vi "Secondary Ball Management and Shoot.vi"   [LabVIEW 2011]
uses:
  Team Code/Robot Global Data.vi
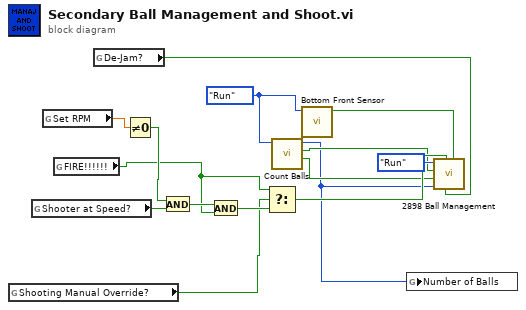
[diagram p0: block diagram]
diagram:
  w1 = enum16{"Init", "Run", "End"}."Run" ("Enum")
  n1 = global read "Robot Global Data.vi" "Shooting Manual Override?"() -> (w9:bool)
  n2 = global read "Robot Global Data.vi" "Shooter at Speed?"() -> (w15:bool)
  n3 = global read "Robot Global Data.vi" "Set RPM"() -> (w12:dbl)
  n4 = global read "Robot Global Data.vi" "FIRE!!!!!!"() -> (w10:bool)
  n5 = global read "Robot Global Data.vi" "De-Jam?"() -> (w3:bool)
  n6 = Not Equal To 0?(x=w12) -> (x != 0?=w11:bool)
  n7 = And(x=w11, y=w15) -> (x .and. y?=w14:bool)
  n8 = And(x=w14, y=w10) -> (x .and. y?=w13:bool)
  n9 = Select(t=w10, s=w9, f=w13) -> (s? t:f=w8:bool)
  n10 = call "Count Balls.vi"("Mode"=w1) -> ("Top Sensor?"=w5:bool, "Bottom Back?"=w6:bool, "Number Of Balls"=w4:i32)  [unwired: 8 in]
  n11 = call "Bottom Front Sensor.vi"("Enum"=w1) -> ("Bottom Front"=w2:bool)  [unwired: 10 in]
  n12 = global write "Robot Global Data.vi" "Number of Balls"(w4) -> ()
  n13 = call "2898 Ball Management.vi"("Bottom Front Sensor"=w2, "De-Jam"=w3, "Shoot?"=w8, "# of Balls"=w4, "Top Ball Sensor"=w5, "Bottom Back Sensor"=w6, "Enum"=enum16{"Init", "Run", "End"}."Run") -> ()  [unwired: 5 in]
